vi "Stop Core.vi"(10 "final error code":i32, 11 "IObserver in":refnum<class "IObserver.lvclass">) -> (3 "IObserver out":refnum<class "IObserver.lvclass">)   [LabVIEW 2017, in "IObserver.lvlib" / "IObserver.lvclass"]
doc: "(<B>Filename</B>: Actor Framework.lvlib:Actor.lvclass:Stop Core.vi)\n\nDefines what the actor does before it stops. Use the <B>final error code</B> input to determine whether the actor shut down in response to an error.\n\nBy default, this method does nothing. A descendant class may override it to define behavior, such as shutting down any processes the actor initiated in its override of the Actor Core method."
uses:
  IObserver.lvclass
  <vilib>/ActorFramework/Actor/Actor.lvclass
  gpm_packages/@cs/event-logger/Source/Composed Log/Types/Log Level.ctl
  gpm_packages/@cs/event-logger/Source/Composed Log/Composed Log.lvlib
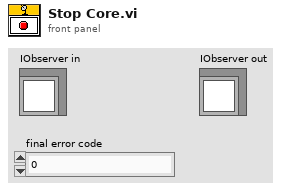
[diagram p1: front panel]
types:
  T1 = typedef "Composed Log.lvlib/Log Level.ctl" = enum16{"Debug", "Info", "Warning", "Error", "Critical"}
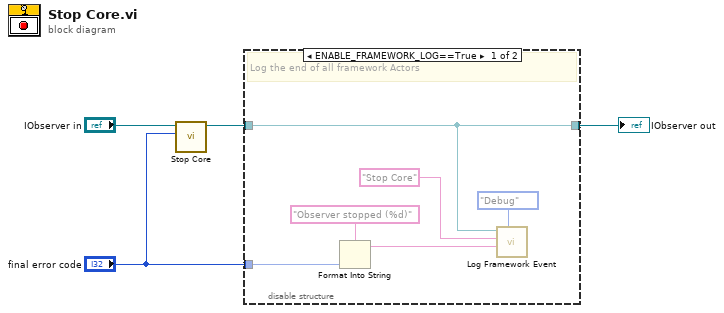
[diagram p0: block diagram]
diagram:
  n1 = call-parent "Stop Core.vi"("final error code"="final error code", "Actor in"="IObserver in") -> ("Actor out"=w3:refnum<class "IObserver.lvclass">)  [unwired: 9 in]
  n2 = disable-structure shown="ENABLE_FRAMEWORK_LOG==True" {
    disable-tunnel: w3 -> [w6 w11]
    disable-tunnel: [w6 w11] -> w2
    disable-tunnel: "final error code" -> [w9 _]
    frame condition #0 {
      # "Log the end of all framework Actors"
      n3 = Format Into String(format string="Observer stopped (%d)", w9) -> (resulting string=w7:string)  [unwired: 2 in, 1 out]
      n4 = call "Log Framework Event.vi"("Event Level (Debug)"=Log_Level."Debug" ("Event Level"), "Data To Log"=w7, "Caller Info (\"\")"="Stop Core" ("Caller Info (\"\")"), "IObserver in"=w6) -> ()  [unwired: 7 in, 1 out]
    }
    frame condition #1 (active) {
      # "Remove all logging from this method at compile time"
    }
  }
  "IObserver out" <- w2
